vi "NI VeriStand - Get Multiple Parameter Values.vi"(7 "Target":string, 8 "error in (no error)":errorcluster, 10 "Parameters":string[](array[string]), 11 "ModelManager in":T1) -> (0 "error out":errorcluster, 2 "Values":dbl[](array[numeric]), 3 "ModelManager out":T1)   [LabVIEW 2020, in "NI_VS ModelManager ExecutionAPI.lvlib"]
doc: "Returns values of model parameters present on the target. You must manually select the polymorphic instance to use."
uses:
  <vilib>/NI VeriStand/Execution/ModelManager/NI_VS ModelManager ExecutionAPI.lvlib
  <vilib>/NI VeriStand/Execution/ModelManager/ModelManagerAPI.ctl
  NationalInstruments.VeriStand.ClientAPI
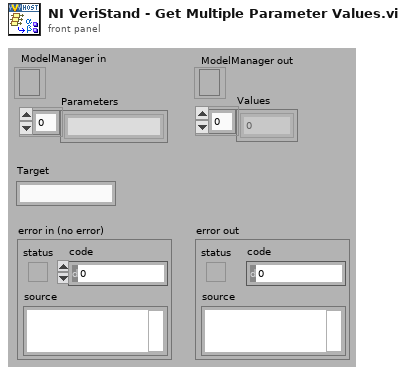
[diagram p1: front panel]
types:
  T1 = typedef "NI_VS ModelManager ExecutionAPI.lvlib/ModelManagerAPI.ctl" = refnum<k24>
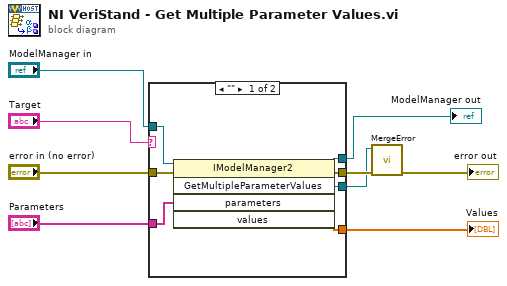
[diagram p0: block diagram]
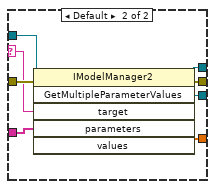
[diagram p2: hidden frame]
diagram:
  n1 = case shown="\"\"" "Target" {
    selector: "Target" -> [_ w19]
    tunnel: "ModelManager in" -> [w16 w24]
    tunnel: [w15 w23] -> w8
    tunnel: "error in (no error)" -> [w14 w22]
    tunnel: [w10 w17] -> w3
    tunnel: "Parameters" -> [w13 w20]
    tunnel: [w12 w21] -> w5
    tunnel: [w11 w18] -> w2
    frame "" {
      n2 = invoke class="IModelManager2" method="GetMultipleParameterValues"(reference=w16, error in=w14, "parameters"=w13) -> (reference out=w15:T1, error out=w10:errorcluster, "GetMultipleParameterValues"=w11:refnum<k24>, "values"=w12:dbl[])  [unwired: 2 in, 1 out]
    }
    frame Default {
      n3 = invoke class="IModelManager2" method="GetMultipleParameterValues"(reference=w24, error in=w22, "target"=w19, "parameters"=w20) -> (reference out=w23:T1, error out=w17:errorcluster, "GetMultipleParameterValues"=w18:refnum<k24>, "values"=w21:dbl[])  [unwired: 2 in, 2 out]
    }
  }
  "ModelManager out" <- w8
  "Values" <- w5
  n4 = call <vilib>:"MergeError.vi"("error in (no error)"=w3, "Error"=w2) -> ("error out"=→"error out":errorcluster)  [unwired: 9 out]
